vi "Adder1.vi"() -> (8 "Adder1":refnum<class "Adder1.lvclass">)   [LabVIEW 2017, in "Adder1.lvclass"]
uses:
  Adder1.lvclass
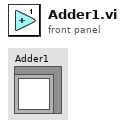
[diagram p1: front panel]
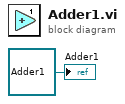
[diagram p0: block diagram]
diagram:
  "Adder1" <- refnum<class "Adder1.lvclass"> refnum ("Adder1.lvclass")
